vi "PD controller.vi"() -> ()   [LabVIEW 2009]
panel:
  out "MV":dbl
  in  "process variable":dbl
  in  "setpoint":dbl
  in  "gain parameters":cluster{"P":dbl, "I":dbl, "D":dbl}
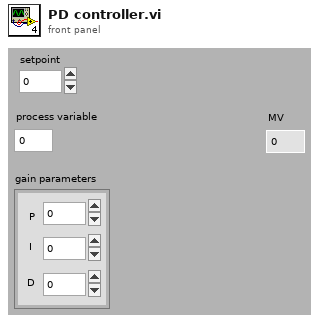
[diagram p1: front panel]
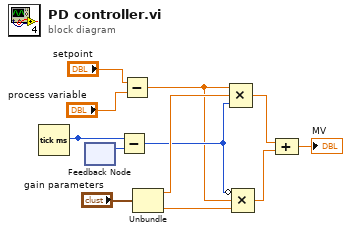
[diagram p0: block diagram]
diagram:
  n1 = Tick Count (ms)() -> (millisecond timer value=w9:u32)
  n2 = feedback #1() -> (w10:u32)  [unwired: 1 in]
  n3 = Subtract(x=w9, y=w10) -> (x-y=w5:u32)
  n4 = Subtract(x="setpoint", y="process variable") -> (x-y=w4:dbl)
  n5 = Unbundle("gain parameters") -> ("P"=w8:dbl, "D"=w6:dbl)  [unwired: 1 out]
  n6 = Compound Arithmetic op=MULTIPLY(w4, w8, w5) -> (w3:dbl)
  n7 = Compound Arithmetic op=MULTIPLY(invert w5, w4, w6) -> (w2:dbl)
  n8 = Compound Arithmetic op=ADD(w3, w2) -> (→"MV":dbl)
